vi "createEvents.vi"(8 "error in (no error)":errorcluster, 11 "SettingsEventsManager in":refnum<class "SettingsEventsManager.lvclass">) -> (0 "error out":errorcluster, 3 "SettingsEventsManager out":refnum<class "SettingsEventsManager.lvclass">)   [LabVIEW 2011, in "Tools.lvlib" / "Settings.lvlib" / "SettingsEventsManager.lvclass"]
uses:
  SettingsEventsManager.lvclass
  SettingsEventsManager.lvclass/SettingsEventsManager.ctl
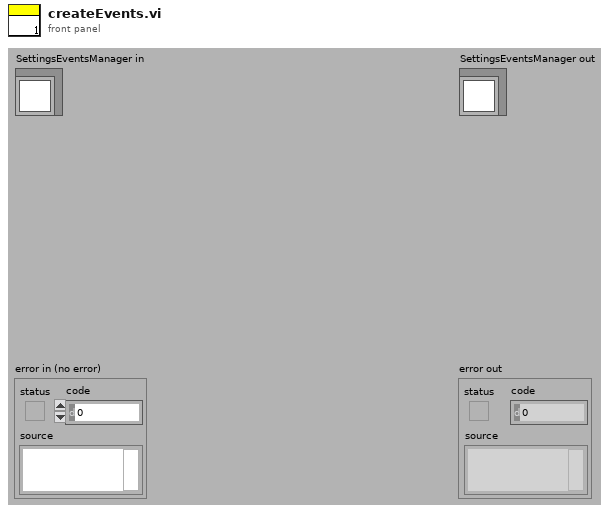
[diagram p1: front panel]
types:
  T1 = cluster{"settingsFrontEndEvents":cluster{"loadSettingsFromPath":refnum<user-event>, "lookUpElementEvent":refnum<user-event>, "saveSettings":refnum<user-event>, "loadSettings":refnum<user-event>, "close":refnum<user-event>, "replaceElement":refnum<user-event>, "findParentNodes":refnum<user-event>, "createNode":refnum<user-event>}, "settingBackEndEvents":cluster{"defaultSettingsPathRequest":refnum<user-event>, "searchResultEvent":refnum<user-event>, "settingsSaved":refnum<user-event>, "settingsLoaded":refnum<user-event>, "foundParentNode":refnum<user-event>}}
  T2 = cluster{"loadSettingsFromPath":cluster{"Path":path}, "lookUpElementEvent":cluster{"lookUpElement":string, "lookUpInElement":string, "typeEnum":enum16{"Number", "String", "NumberArray", "StringArray", "xmlNode"}}, "saveSettings":cluster{"Path":path}, "loadSettings":cluster{"Dummy":bool}, "close":cluster{"dummy":bool}, "replaceElement":cluster{"replaceElement":string, "replaceInElement":string, "replaceWithValue":string}, "findParentNodes":cluster{"searchElement":string, "type":enum16{"element", "attribute", "value"}, "searchIn":string}, "createNode":cluster{"xmlNodeString":string, "createInNodePath":string}}
  T3 = cluster{"defaultSettingsPathRequest":cluster{"Path":path}, "searchResultEvent":cluster{"elementName":string, "typeEnum":enum16{"Number", "String", "NumberArray", "StringArray", "xmlNode"}, "dataElement":variant, "lookedUpInElement":string}, "settingsSaved":cluster{"Path":path}, "settingsLoaded":cluster{"Dummy":bool}, "foundParentNode":cluster{"Paths":string[], "searchElement":string, "type":enum16{"element", "attribute", "value"}, "searchIn":string}}
  T4 = cluster{"elementName":string, "typeEnum":enum16{"Number", "String", "NumberArray", "StringArray", "xmlNode"}, "dataElement":variant, "lookedUpInElement":string}
  T5 = cluster{"Paths":string[], "searchElement":string, "type":enum16{"element", "attribute", "value"}, "searchIn":string}
  T6 = cluster{"lookUpElement":string, "lookUpInElement":string, "typeEnum":enum16{"Number", "String", "NumberArray", "StringArray", "xmlNode"}}
  T7 = cluster{"replaceElement":string, "replaceInElement":string, "replaceWithValue":string}
  T8 = cluster{"searchElement":string, "type":enum16{"element", "attribute", "value"}, "searchIn":string}
  T9 = cluster{"xmlNodeString":string, "createInNodePath":string}
  T10 = cluster{"defaultSettingsPathRequest":refnum<user-event>, "searchResultEvent":refnum<user-event>, "settingsSaved":refnum<user-event>, "settingsLoaded":refnum<user-event>, "foundParentNode":refnum<user-event>}
  T11 = cluster{"loadSettingsFromPath":refnum<user-event>, "lookUpElementEvent":refnum<user-event>, "saveSettings":refnum<user-event>, "loadSettings":refnum<user-event>, "close":refnum<user-event>, "replaceElement":refnum<user-event>, "findParentNodes":refnum<user-event>, "createNode":refnum<user-event>}
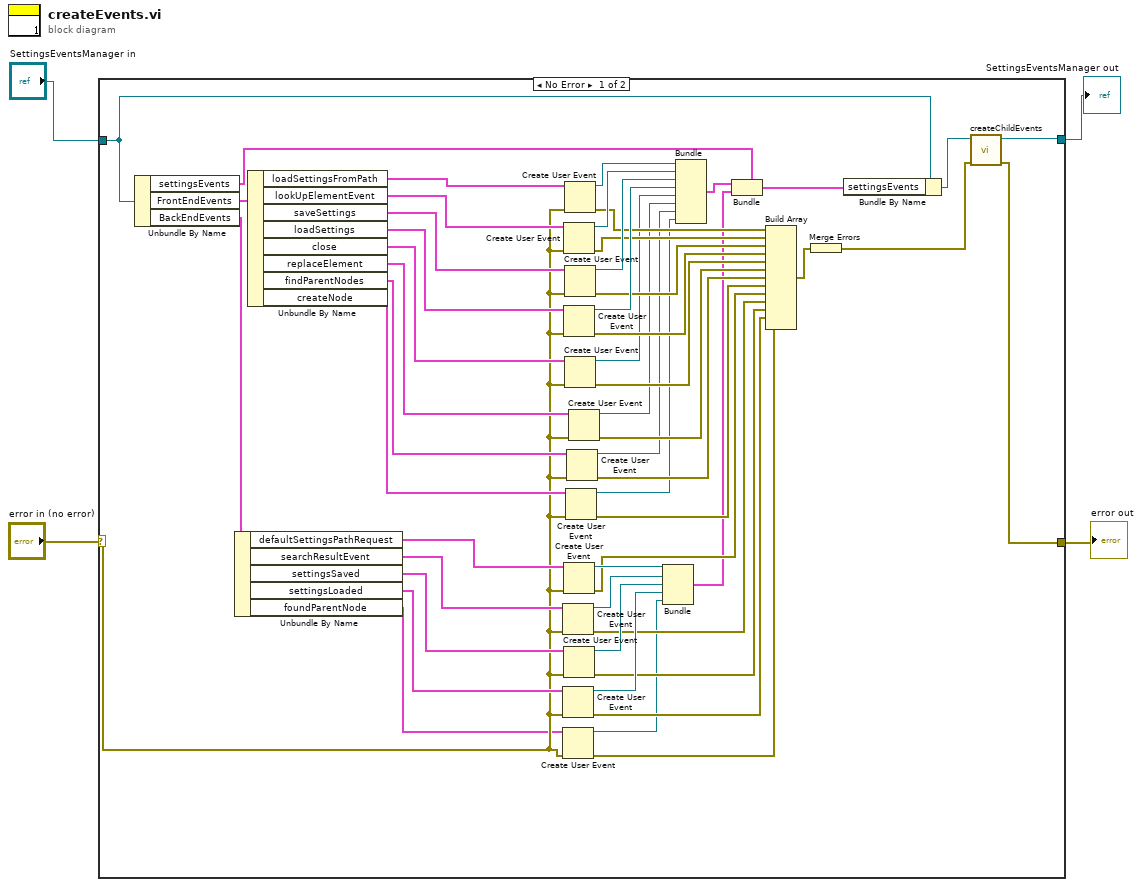
[diagram p0: block diagram]
diagram:
  n1 = case shown="No Error" "error in (no error)" {
    selector: "error in (no error)" -> [w14 w58]
    tunnel: [w26 w58] -> w3
    tunnel: [w25 w57] -> w1
    tunnel: "SettingsEventsManager in" -> [w54 w57]
    frame No Error {
      n2 = Unbundle By Name(w54) -> ("settingsEvents"=w8:T1, "FrontEndEvents"=w30:T2, "BackEndEvents"=w29:T3)
      n3 = Unbundle By Name(w29) -> ("defaultSettingsPathRequest"=w47:cluster{"Path":path}, "searchResultEvent"=w46:T4, "settingsSaved"=w45:cluster{"Path":path}, "settingsLoaded"=w44:cluster{"Dummy":bool}, "foundParentNode"=w13:T5)
      n4 = Unbundle By Name(w30) -> ("loadSettingsFromPath"=w53:cluster{"Path":path}, "lookUpElementEvent"=w52:T6, "saveSettings"=w51:cluster{"Path":path}, "loadSettings"=w50:cluster{"Dummy":bool}, "close"=w24:cluster{"dummy":bool}, "replaceElement"=w21:T7, "findParentNodes"=w18:T8, "createNode"=w17:T9)
      n5 = Create User Event(user event datatype=w46, error in=w14) -> (user event=w41:refnum<user-event>, error out=w34:errorcluster)
      n6 = Create User Event(user event datatype=w44, error in=w14) -> (user event=w43:refnum<user-event>, error out=w32:errorcluster)
      n7 = Create User Event(user event datatype=w13, error in=w14) -> (user event=w9:refnum<user-event>, error out=w12:errorcluster)
      n8 = Create User Event(user event datatype=w52, error in=w14) -> (user event=w55:refnum<user-event>, error out=w38:errorcluster)
      n9 = Create User Event(user event datatype=w50, error in=w14) -> (user event=w48:refnum<user-event>, error out=w36:errorcluster)
      n10 = Create User Event(user event datatype=w47, error in=w14) -> (user event=w40:refnum<user-event>, error out=w35:errorcluster)
      n11 = Create User Event(user event datatype=w45, error in=w14) -> (user event=w42:refnum<user-event>, error out=w33:errorcluster)
      n12 = Create User Event(user event datatype=w53, error in=w14) -> (user event=w56:refnum<user-event>, error out=w39:errorcluster)
      n13 = Create User Event(user event datatype=w51, error in=w14) -> (user event=w49:refnum<user-event>, error out=w37:errorcluster)
      n14 = Create User Event(user event datatype=w24, error in=w14) -> (user event=w22:refnum<user-event>, error out=w23:errorcluster)
      n15 = Create User Event(user event datatype=w17, error in=w14) -> (user event=w10:refnum<user-event>, error out=w15:errorcluster)
      n16 = Create User Event(user event datatype=w18, error in=w14) -> (user event=w11:refnum<user-event>, error out=w16:errorcluster)
      n17 = Create User Event(user event datatype=w21, error in=w14) -> (user event=w19:refnum<user-event>, error out=w20:errorcluster)
      n18 = Bundle("defaultSettingsPathRequest"=w40, "searchResultEvent"=w41, "settingsSaved"=w42, "settingsLoaded"=w43, "foundParentNode"=w9) -> (w5:T10)  [unwired: 1 in]
      n19 = Bundle("loadSettingsFromPath"=w56, "lookUpElementEvent"=w55, "saveSettings"=w49, "loadSettings"=w48, "close"=w22, "replaceElement"=w19, "findParentNodes"=w11, "createNode"=w10) -> (w6:T11)  [unwired: 1 in]
      n20 = Bundle(cluster=w8, "settingsFrontEndEvents"=w6, "settingBackEndEvents"=w5) -> (w7:T1)
      n21 = Build Array(w39, w38, w37, w36, w23, w20, w16, w15, w35, w34, w33, w32, w12) -> (w31:errorcluster[])
      n22 = Merge Errors(w31) -> (w27:errorcluster)
      n23 = Bundle By Name(cluster=w54, "settingsEvents"=w7) -> (w28:refnum<class "SettingsEventsManager.lvclass">)
      n24 = call-dynamic "createChildEvents.vi"("error in (no error)"=w27, "SettingsEventsManager in"=w28) -> ("error out"=w26:errorcluster, "SettingsEventsManager out"=w25:refnum<class "SettingsEventsManager.lvclass">)  [unwired: 8 in]
    }
    frame Error {
    }
  }
  "error out" <- w3
  "SettingsEventsManager out" <- w1
